vi "Intan_PauseDatastream.vi"(3 "error in":errorcluster, 5 "VISA resource name":refnum<visa-resource-name>="COM1") -> (0 "error out":errorcluster, 1 "Text response":string, 2 "VISA resource name out":refnum<visa-resource-name>)   [LabVIEW 2011]
doc: "Use this VI to pause the data stream. This pauses the ADC convert commands and serial.write() commands. The data stream can resume using the StartDataStream.vi"
panel:
  in  "event char (reserved char in Teensyduino code)":string="p"
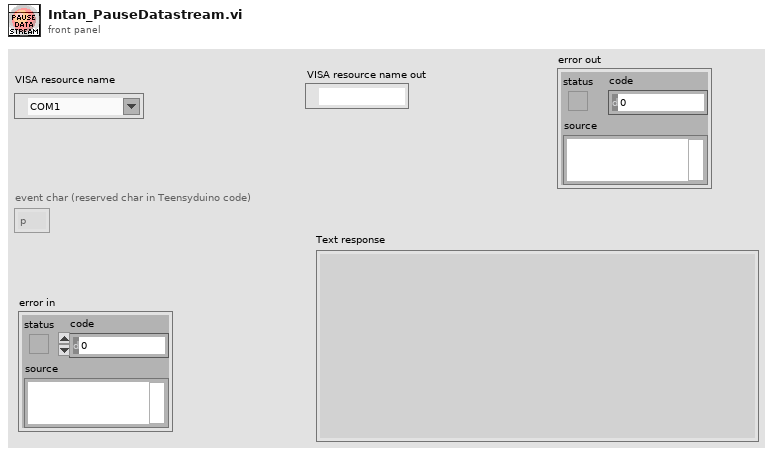
[diagram p1: front panel]
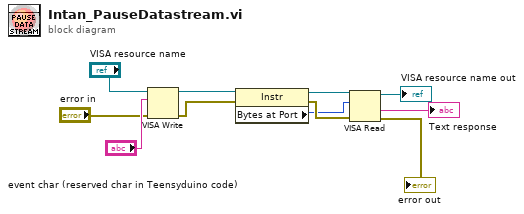
[diagram p0: block diagram]
diagram:
  n1 = VISA Write(VISA resource name="VISA resource name", write buffer="event char (reserved char in Teensyduino code)", error in (no error)="error in") -> (VISA resource name out=w3:refnum<visa-resource-name>, error out=w2:errorcluster)  [unwired: 1 out]
  n2 = property class="Instr"(reference=w3, error in=w2) -> (reference out=w9:refnum<visa-resource-name>, error out=w8:errorcluster, "Bytes at Port"=w7:u32)
  n3 = VISA Read(VISA resource name=w9, byte count=w7, error in (no error)=w8) -> (VISA resource name out=→"VISA resource name out":refnum<visa-resource-name>, read buffer=→"Text response":string, error out=→"error out":errorcluster)  [unwired: 1 out]
